vi "Clear Views.vi"(8 "error in (no error)":errorcluster, 11 "Main In":refnum<class "Main.lvclass">) -> (0 "error out":errorcluster, 3 "Main Out":refnum<class "Main.lvclass">)   [LabVIEW 2020, in "Main.lvclass"]
uses:
  Main.lvclass
  Debug View/Debug View.lvclass
  Main.lvclass/Main.ctl
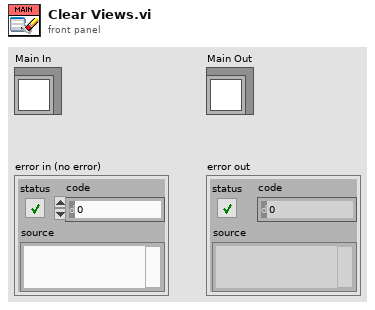
[diagram p1: front panel]
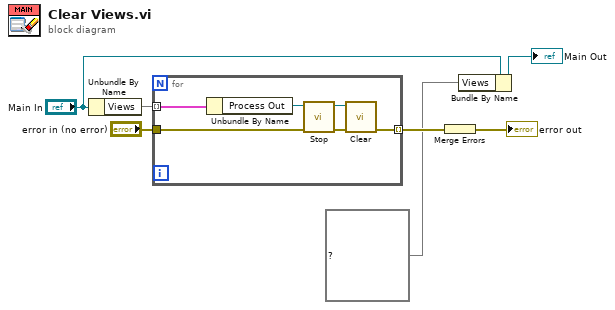
[diagram p0: block diagram]
diagram:
  n1 = Unbundle By Name("Main In") -> ("Views"=w7:map{string, refnum<class "Debug View.lvclass">})
  n2 = for {
    tunnel: w7 -> [w13] mode=indexing
    tunnel: "error in (no error)" -> [w9]
    tunnel: [w8] -> w4 mode=indexing
    n3 = Unbundle By Name(w13) -> ("Process Out"=w10:refnum<class "Debug View.lvclass">)
    n4 = call "Stop.vi"("error in (no error)"=w9, "Process In"=w10) -> ("error out"=w11:errorcluster, "Process Out"=w12:refnum<class "Debug View.lvclass">)  [unwired: 8 in]
    n5 = call-dynamic "Clear.vi"("error in (no error)"=w11, "Debug View In"=w12) -> ("error out"=w8:errorcluster)  [unwired: 9 in]
  }
  n6 = Merge Errors(w4) -> (→"error out":errorcluster)
  n7 = Bundle By Name(cluster="Main In", "Views"=map{string, refnum<class "Debug View.lvclass">} {}) -> (→"Main Out":refnum<class "Main.lvclass">)
